vi "Legend VI.vi"(3 "Legend in":cluster{"Color Box":u32, "String":string}[](array[cluster]), 4 "Legend Ref in":refnum<vi>) -> (1 "Legend Ref out":refnum<vi>)   [LabVIEW 2018]
doc: "Restructures the 1D legend array as a 2D legend and writes it to the front panel"
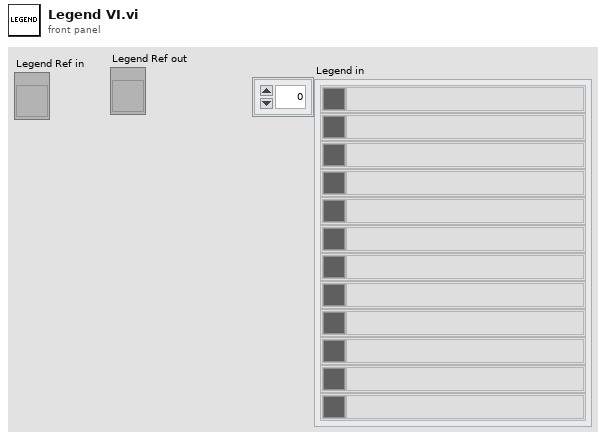
[diagram p1: front panel]
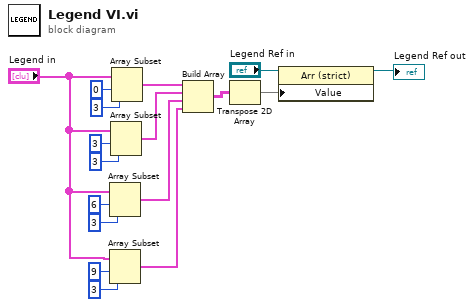
[diagram p0: block diagram]
diagram:
  n1 = Array Subset(array="Legend in", index=6, length=3) -> (w5:cluster{"Color Box":u32, "String":string}[])
  n2 = Array Subset(array="Legend in", index=9, length=3) -> (w1:cluster{"Color Box":u32, "String":string}[])
  n3 = Array Subset(array="Legend in", index=3, length=3) -> (w13:cluster{"Color Box":u32, "String":string}[])
  n4 = Array Subset(array="Legend in", index=0, length=3) -> (w12:cluster{"Color Box":u32, "String":string}[])
  n5 = Build Array(w12, w13, w5, w1) -> (w17:cluster{"Color Box":u32, "String":string}[][])
  n6 = Transpose 2D Array(2D array=w17) -> (transposed array=w15:cluster{"Color Box":u32, "String":string}[][])
  n7 = property class="Arr (strict)"(reference="Legend Ref in", "Value"=w15) -> (reference out=→"Legend Ref out":refnum<vi>)  [unwired: 1 in, 1 out]
